vi "MyGlobal.vi"() -> ()   [LabVIEW 2017]
uses:
  MyGlobal-Global.vi
panel:
  in  "布尔 2":bool
  out "布尔":bool
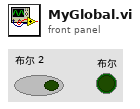
[diagram p1: front panel]
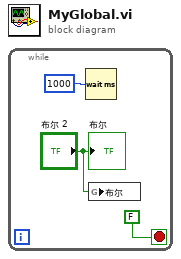
[diagram p0: block diagram]
diagram:
  n1 = while {
    stop <- FALSE stop-if-true
    n2 = Wait (ms)(milliseconds to wait=u32 1000 ("等待时间（毫秒）")) -> ()  [unwired: 1 out]
    n3 = global write "MyGlobal-Global.vi" "布尔"("布尔 2") -> ()
    "布尔" <- "布尔 2"
  }
